vi "niusrprios Self Measure Rx IQ Offset.vi"(0 "niUsrpRio Session":T1={"FPGA Interface"=refnum, "RIO Interface Number"=0, "Data Clock Rate"=0, "FPGA Data Clock Rate"=0, "Global Settings Register Bus"=refnum, "Radio 0 Settings Register Bus"=refnum, "Radio 1 Settings Register Bus"=refnum, "Radio Settings Bus Semaphore"=refnum, "DB Queues"=[], "Characterization Data Valid?"=FALSE, "EEPROM Header"={"Checksum"=0, "Product Code"=0, "Hardware Current Version"=0, "Hardware Oldest Compatible Version"=0, "EEPROM Map Current Version"=0, "EEPROM Map Oldest Compatible Version"=0, "User Password"="", "Pointer to Factory Header"=0, "Pointer to User Header"=0, "Recommended Interval"=0, "Number of Reserved Bytes"=9, "Number of Daughterboards"=0, "Daughterboard IDs"=[], "Daughterboard Serial Numbers"=[]}, "Device Data Header"={"Checksum"=0, "Number of Channels"=0, "Number of Gain Settings"=[], "Pointer to Characterization Data"=[], "Number of Reserved Bytes"=27, "Number of Frequencies"=[]}, "EEPROM Characterization Header"={"Checksum"=0, "Date"=timestamp(0 s since 1904-01-01), "Temperature"=0.0, "Misc. Info"="", "Pointer to Device Data Header"=0, "Number of Reserved Bytes"=28}, "Characterization Data"=[], "FPGA Current Version"=0, "FPGA Oldest Compatible Version"=0, "Fixed Logic Current Version"=0, "Fixed Logic Oldest Compatible Version"=0, "FPGA Radio Settings Bus Current Version"=0, "FPGA Radio Settings Bus Oldest Compatible Version"=0, "FPGA Board Config Current Version"=0, "FPGA Board Config Oldest Compatible Version"=0, "Daughterboard Clock Rate"=0} {"Daughterboard Clock Rate" format="%#.3pHz"; "FPGA Data Clock Rate" format="%#.3pHz"; "Data Clock Rate" format="%#.3pHz"; "Characterization Data"."Frequencies [Hz]" format="%#_6p"; "EEPROM Characterization Header"."Pointer to Device Data Header" format="%x"; "EEPROM Characterization Header"."Checksum" format="%x"; "Device Data Header"."Pointer to Characterization Data" format="%x"; "Device Data Header"."Checksum" format="%x"; "EEPROM Header"."Pointer to User Header" format="%x"; "EEPROM Header"."Pointer to Factory Header" format="%x"; "EEPROM Header"."Product Code" format="%x"; "EEPROM Header"."Checksum" format="%x"}, 1 "channel":string(combo)="rx/RF 0", 5 "carrier freq":dbl=2400000000.0 format="%#_6p", 7 "IQ rate":dbl=10000000.0 format="%#_6p", 9 "gain":dbl=15.0 format="%#_6f", 11 "error in (no error)":errorcluster, 12 "tuning settle (ms)":u32=100, 13 "number of samples":u32=10000, 14 "transient samples to throw out":u32=4000) -> (3 "offset":cdb, 4 "niUsrpRio Session (out)":T1={"FPGA Interface"=refnum, "RIO Interface Number"=0, "Data Clock Rate"=0, "FPGA Data Clock Rate"=0, "Global Settings Register Bus"=refnum, "Radio 0 Settings Register Bus"=refnum, "Radio 1 Settings Register Bus"=refnum, "Radio Settings Bus Semaphore"=refnum, "DB Queues"=[], "Characterization Data Valid?"=FALSE, "EEPROM Header"={"Checksum"=0, "Product Code"=0, "Hardware Current Version"=0, "Hardware Oldest Compatible Version"=0, "EEPROM Map Current Version"=0, "EEPROM Map Oldest Compatible Version"=0, "User Password"="", "Pointer to Factory Header"=0, "Pointer to User Header"=0, "Recommended Interval"=0, "Number of Reserved Bytes"=9, "Number of Daughterboards"=0, "Daughterboard IDs"=[], "Daughterboard Serial Numbers"=[]}, "Device Data Header"={"Checksum"=0, "Number of Channels"=0, "Number of Gain Settings"=[], "Pointer to Characterization Data"=[], "Number of Reserved Bytes"=27, "Number of Frequencies"=[]}, "EEPROM Characterization Header"={"Checksum"=0, "Date"=timestamp(0 s since 1904-01-01), "Temperature"=0.0, "Misc. Info"="", "Pointer to Device Data Header"=0, "Number of Reserved Bytes"=28}, "Characterization Data"=[], "FPGA Current Version"=0, "FPGA Oldest Compatible Version"=0, "Fixed Logic Current Version"=0, "Fixed Logic Oldest Compatible Version"=0, "FPGA Radio Settings Bus Current Version"=0, "FPGA Radio Settings Bus Oldest Compatible Version"=0, "FPGA Board Config Current Version"=0, "FPGA Board Config Oldest Compatible Version"=0, "Daughterboard Clock Rate"=0} {"Daughterboard Clock Rate" format="%#.3pHz"; "FPGA Data Clock Rate" format="%#.3pHz"; "Data Clock Rate" format="%#.3pHz"; "Characterization Data"."Frequencies [Hz]" format="%#_6p"; "EEPROM Characterization Header"."Pointer to Device Data Header" format="%x"; "EEPROM Characterization Header"."Checksum" format="%x"; "Device Data Header"."Pointer to Characterization Data" format="%x"; "Device Data Header"."Checksum" format="%x"; "EEPROM Header"."Pointer to User Header" format="%x"; "EEPROM Header"."Pointer to Factory Header" format="%x"; "EEPROM Header"."Product Code" format="%x"; "EEPROM Header"."Checksum" format="%x"}, 6 "coerced frequency":dbl format="%#_6p", 15 "error out":errorcluster)   [LabVIEW 2015]
uses:
  <instrlib>/niUsrpRio/Config/v1/Host/Public/niUsrpRio Session.ctl
  <instrlib>/_niInstr/Register Bus/v0/Host/Public/Register Bus Session.ctl
  <instrlib>/_niInstr/Register Bus/v0/Host/Private/Session Data.ctl
  <instrlib>/niUsrpRio/Config/v1/Host/Private/DB Queue Reference.ctl
  <instrlib>/niUsrpRio/Config/v1/Host/Private/Daughterboard Data.ctl
  <instrlib>/niUsrpRio/Config/v1/Host/Private/ATR state data.ctl
  <instrlib>/niUsrpRio/Config/v1/Host/Private/Antenna Configuration.ctl
  <instrlib>/niUsrpRio/Config/v1/Host/Private/CPLD Power Mode.ctl
  <instrlib>/niUsrpRio/Config/v1/Host/Public/EEPROM Header.ctl
  <instrlib>/niUsrpRio/Config/v1/Host/Public/EEPROM Device Data Header.ctl
  <instrlib>/niUsrpRio/Config/v1/Host/Public/EEPROM Characterization Header.ctl
  <instrlib>/niUsrpRio/Config/v1/Host/Public/Characterization Data.ctl
  <instrlib>/niUsrpRio/Config/v1/Host/Public/IQ Imbalance.ctl
  niusrprios Streaming Xvcr FPGA Ref.ctl
  <instrlib>/niUsrpRio/Config/v1/Host/Public/What to Wait for.ctl
  <vilib>/Analysis/baseanly.llb/Mean (CDB).vi
  niusrprios Fetch Rx Data (CDB WDT).vi
  <vilib>/rvi/errors/niLvFpgaAdjustHostInterfaceError.vi
  <vilib>/Utility/error.llb/Error Cluster From Error Code.vi
  <vilib>/rvi/interface/nirviReadWriteControl/nirviReadWriteControl.xnode
  <instrlib>/niUsrpRio/Config/v1/Host/niUsrpRio Config v1 Host.lvlib
  <vilib>/Analysis/NI_AALBase.lvlib
  NiFpgaLv.dll
  <vilib>/rvi/interface/Simulation/niFpgaSimulationCallBeginRW.vi
  <instrlib>/_niInstr/Register Bus/v0/Host/niInstr Register Bus v0 Host.lvlib
panel:
  out "Waveform Graph":waveform(dbl)[](graph)
  in  "Active Antenna":string(combo)="RX1"
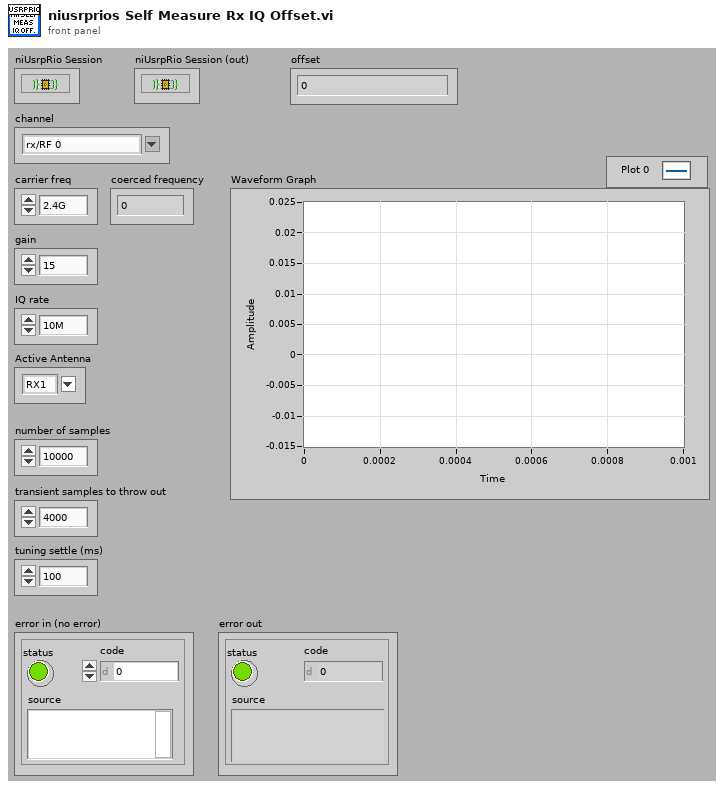
[diagram p1: front panel]
types:
  T1 = typedef "niUsrpRio Config v1 Host.lvlib/niUsrpRio Session.ctl" = cluster{"FPGA Interface":refnum<k20>, "RIO Interface Number":u32, "Data Clock Rate":u32, "FPGA Data Clock Rate":u32, "Global Settings Register Bus":T2, "Radio 0 Settings Register Bus":T2, "Radio 1 Settings Register Bus":T2, "Radio Settings Bus Semaphore":T3, "DB Queues":T4[], "Characterization Data Valid?":bool, "EEPROM Header":T5, "Device Data Header":T6, "EEPROM Characterization Header":T7, "Characterization Data":T8[], "FPGA Current Version":u32, "FPGA Oldest Compatible Version":u32, "Fixed Logic Current Version":u32, "Fixed Logic Oldest Compatible Version":u32, "FPGA Radio Settings Bus Current Version":u32, "FPGA Radio Settings Bus Oldest Compatible Version":u32, "FPGA Board Config Current Version":u32, "FPGA Board Config Oldest Compatible Version":u32, "Daughterboard Clock Rate":u32}
  T2 = typedef "niInstr Register Bus v0 Host.lvlib/Register Bus Session.ctl" = refnum<queue>
  T3 = typedef "Semaphore RefNum" = refnum<k1>
  T4 = typedef "niUsrpRio Config v1 Host.lvlib/DB Queue Reference.ctl" = refnum<queue>
  T5 = typedef "niUsrpRio Config v1 Host.lvlib/EEPROM Header.ctl" = cluster{"Checksum":u32, "Product Code":u16, "Hardware Current Version":u16, "Hardware Oldest Compatible Version":u16, "EEPROM Map Current Version":u16, "EEPROM Map Oldest Compatible Version":u16, "User Password":string, "Pointer to Factory Header":u32, "Pointer to User Header":u32, "Recommended Interval":u16, "Number of Reserved Bytes":i32, "Number of Daughterboards":u8, "Daughterboard IDs":u16[], "Daughterboard Serial Numbers":string[]}
  T6 = typedef "niUsrpRio Config v1 Host.lvlib/EEPROM Device Data Header.ctl" = cluster{"Checksum":u32, "Number of Channels":u8, "Number of Gain Settings":u16[], "Pointer to Characterization Data":u32[], "Number of Reserved Bytes":i32, "Number of Frequencies":u16[]}
  T7 = typedef "niUsrpRio Config v1 Host.lvlib/EEPROM Characterization Header.ctl" = cluster{"Checksum":u32, "Date":timestamp, "Temperature":sgl, "Misc. Info":string, "Pointer to Device Data Header":u32, "Number of Reserved Bytes":i32}
  T8 = typedef "niUsrpRio Config v1 Host.lvlib/Characterization Data.ctl" = cluster{"Gains[dB]":dbl[], "Frequencies [Hz]":dbl[], "IQ Imbalance Table":T9[], "Measured Gains[dB]":dbl[][]}
  T9 = typedef "niUsrpRio Config v1 Host.lvlib/IQ Imbalance.ctl" = cluster{"Gain Imbalance [linear]":dbl, "Phase Imbalance [radians]":dbl, "Offset":cdb}
  T10 = typedef "niUsrpRio Config v1 Host.lvlib/What to Wait for.ctl" = enum16{"Global Settings SPI Ready", "Radio Clocks Valid", "ADC Clock PLL Locked", "Clock Chip Locked", "LO Locked", "GPS Locked", "DRAM Ready", "GPS NMEA Data Ready", "DAC PLL Locked", "DAC Sync Locked", "ADC Data Valid"}
  T11 = typedef "niusrprios Streaming Xvcr FPGA Ref.ctl" = refnum<k20>
  T12 = cluster{"inline gain I":fxp<+/-,18,1>, "inline gain Q":fxp<+/-,18,1>, "cross gain I":fxp<+/-,18,1>, "cross gain Q":fxp<+/-,18,1>, "pre-gain offset I":fxp<+/-,18,1>, "pre-gain offset Q":fxp<+/-,18,1>, "post-gain offset I":fxp<+/-,18,1>, "post-gain offset Q":fxp<+/-,18,1>}
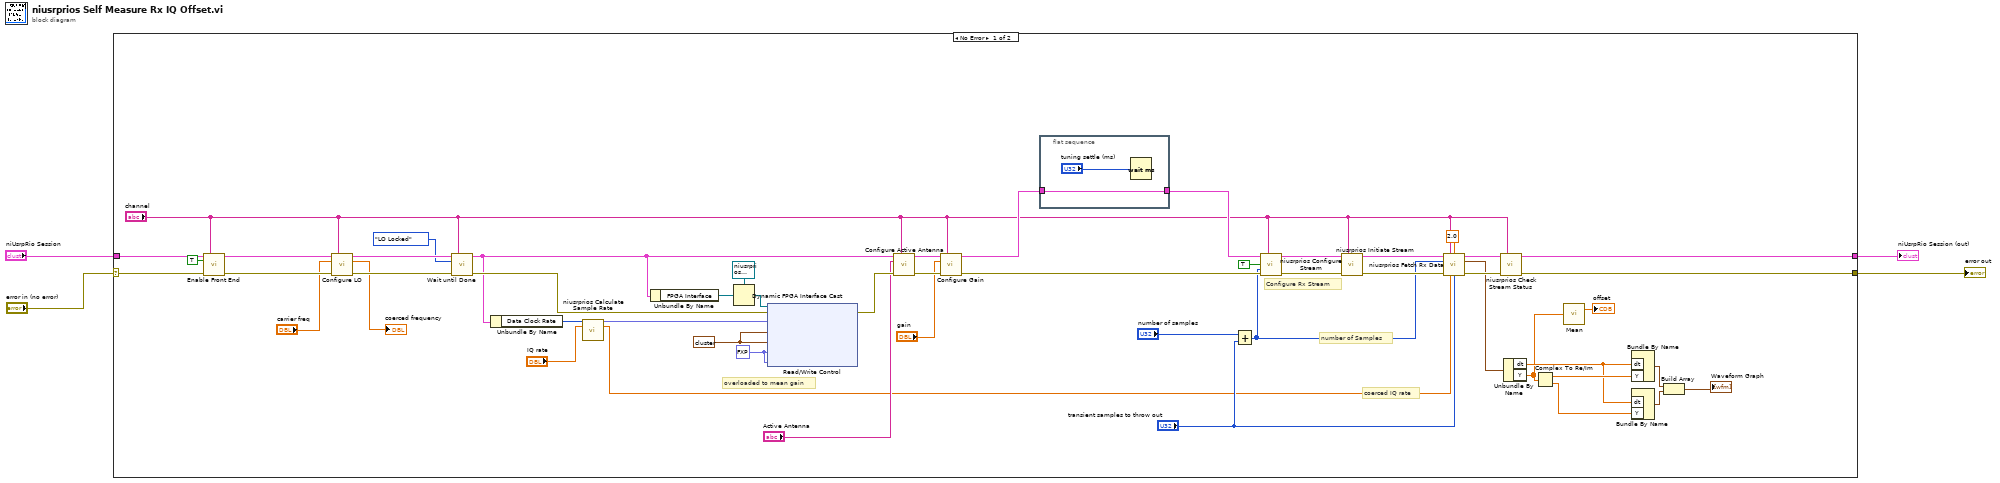
[diagram p0: block diagram]
diagram:
  n1 = case shown="No Error" "error in (no error)" {
    selector: "error in (no error)" -> [w34 w60]
    tunnel: [w18 w60] -> w4
    tunnel: [w17 w59] -> w2
    tunnel: "niUsrpRio Session" -> [w11 w59]
    frame No Error {
      w31 = fxp<+/-,48,0> 0.0 ("rx 0.frequency shift")
      w37 = T12 {"inline gain I"=0.9999923706054688, "inline gain Q"=0.9999923706054688, "cross gain I"=0.0, "cross gain Q"=0.0, "pre-gain offset I"=0.0, "pre-gain offset Q"=0.0, "post-gain offset I"=0.0, "post-gain offset Q"=0.0} ("rx 0.impairments")
      # "overloaded to mean gain"
      # "coerced IQ rate"
      # "number of Samples"
      # "Configure Rx Stream"
      n2 = call <instrlib>:"Enable Front End.vi"("niUsrpRio Session"=w11, "scope"="channel", "enable"=TRUE, "error in"=w34) -> ("niUsrpRio Session (out)"=w32:T1, "error out"=w33:errorcluster)  [unwired: 10 in]
      n3 = call <instrlib>:"Configure LO.vi"("niUsrpRio Session"=w32, "scope"="channel", "frequency"="carrier freq", "Error In"=w33) -> ("niUsrpRio Session (out)"=w43:T1, "coerced frequency"=→"coerced frequency":dbl, "Error Out"=w44:errorcluster)  [unwired: 9 in]
      n4 = call <instrlib>:"Wait until Done.vi"("niUsrpRio Session"=w43, "scope"="channel", "What to Wait for"=What_to_Wait_for."LO Locked", "error in"=w44) -> ("niUsrpRio Session (out)"=w29:T1, "error out"=w30:errorcluster)  [unwired: 10 in]
      n5 = Unbundle By Name(w29) -> ("Data Clock Rate"=w28:u32)
      n6 = call "niusrprios Calculate Sample Rate.vi"("data clock rate"=w28, "sample rate"="IQ rate") -> ("decimation sample rate"=w41:fxp<+,48,1>, "coerced sample rate"=w5:dbl)  [unwired: 12 in]
      n7 = Unbundle By Name(w29) -> ("FPGA Interface"=w45:refnum<k20>)
      n8 = Dynamic FPGA Interface Cast(Session In=T11 refnum ("FPGA VI Reference Out"), Type=w45) -> (Session Out=w46:T11)
      n9 = xnode "Read/Write Control"("FPGA VI Reference In"=w46, "error in"=w30, "rx.output sample rate"=w41, "rx 0.impairments"=w37, "rx 1.impairments"=w37, "rx 0.frequency shift"=w31, "rx 1.frequency shift"=w31) -> ("error out"=w40:errorcluster)  [unwired: 1 out]
      n10 = call <instrlib>:"Configure Active Antenna.vi"("niUsrpRio Session"=w29, "scope"="channel", "active antenna"="Active Antenna", "error in"=w40) -> ("niUsrpRio Session (out)"=w38:T1, "error out"=w39:errorcluster)  [unwired: 9 in, 1 out]
      n11 = call <instrlib>:"Configure Gain.vi"("niUsrpRio Session"=w38, "scope"="channel", "gain"="gain", "Error In"=w39) -> ("niUsrpRio Session (out)"=w53:T1, "Error Out"=w52:errorcluster)  [unwired: 9 in, 1 out]
      n12 = flat-sequence {
        tunnel: w53 -> [w57]
        tunnel: [w57] -> w54
        frame #0 {
          # "Wait for the RF filter to settle.  This can be removed if you are certain the RF filter setting did not change."
          n13 = Wait (ms)(milliseconds to wait="tuning settle (ms)") -> ()  [unwired: 1 out]
        }
      }
      n14 = Add(x="number of samples", y="transient samples to throw out") -> (x+y=w49:u32)
      n15 = call "niusrprios Configure Stream.vi"("niUsrpRio Session"=w54, "scope"="channel", "number of samples is finite"=TRUE ("Number of Samples is Finite"), "number of samples"=w49, "error in"=w52) -> ("niUsrpRio Session (out)"=w51:T1, "error out"=w27:errorcluster)  [unwired: 9 in]
      n16 = call "niusrprios Initiate Stream.vi"("niUsrpRio Session"=w51, "scope"="channel", "error in"=w27) -> ("niUsrpRio Session (out)"=w7:T1, "error out"=w56:errorcluster)  [unwired: 11 in]
      n17 = call-poly "niusrprios Fetch Rx Data.vi"("niUsrpRio Session"=w7, "scope"="channel", "vertical range [Vpp]"=2.0, "number of samples"=w49, "error in"=w56, "sample rate"=w5, "leading samples to trim"="transient samples to throw out") -> ("niUsrpRio Session (out)"=w50:T1, "Waveform"=w20:waveform(cdb), "error out"=w48:errorcluster)  [unwired: 6 in]
      n18 = call "niusrprios Check Stream Status.vi"("niUsrpRio Session"=w50, "scope"="channel", "error in"=w48) -> ("niUsrpRio Session (out)"=w17:T1, "error out"=w18:errorcluster)  [unwired: 10 in, 1 out]
      n19 = Unbundle By Name(w20) -> ("dt"=w22:dbl, "Y"=w19:cdb[])
      n20 = Complex To Re/Im(x + iy=w19) -> (x=w25:dbl[], y=w24:dbl[])
      n21 = call-poly <vilib>:"Mean.vi"("X"=w19) -> ("mean"=→"offset":cdb)  [unwired: 1 out]
      n22 = Bundle By Name("dt"=w22, "Y"=w25) -> (w21:waveform(dbl))  [unwired: 1 in]
      n23 = Bundle By Name("dt"=w22, "Y"=w24) -> (w23:waveform(dbl))  [unwired: 1 in]
      n24 = Build Array(w21, w23) -> (→"Waveform Graph":waveform(dbl)[])
    }
    frame Error {
    }
  }
  "error out" <- w4
  "niUsrpRio Session (out)" <- w2
